vi "Too Big.vi"() -> ()   [LabVIEW 2010]
doc: "This program dispalys a message to the user if the user's parameters cause the Moving Message Board display to be too big for the monitor which it it trying to be displayed on."
panel:
  in  "OK Button":bool
  # "The Moving Message Board\nis too big for the monitor!\n\nPlease adjust LED size and/or\nDisplay size and try again."
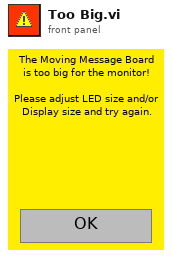
[diagram p1: front panel]
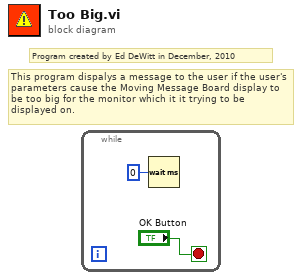
[diagram p0: block diagram]
diagram:
  # "This program dispalys a message to the user if the user's parameters cause the Moving Message Board display to be too big for the monitor which it it trying to be displayed on."
  # "Program created by Ed DeWitt in December, 2010"
  n1 = while {
    stop <- "OK Button" stop-if-true
    n2 = Wait (ms)(milliseconds to wait=u32 0) -> ()  [unwired: 1 out]
  }
